vi "Down.vi"(8 "error in (no error)":errorcluster, 11 "Hijo in":refnum<class "Hijo.lvclass">) -> (0 "error out":errorcluster, 3 "Hijo out":refnum<class "Hijo.lvclass">)   [LabVIEW 2020, in "Hijo.lvlib" / "Hijo.lvclass"]
uses:
  Hijo.lvclass
  Hijo.lvclass/Hijo.ctl
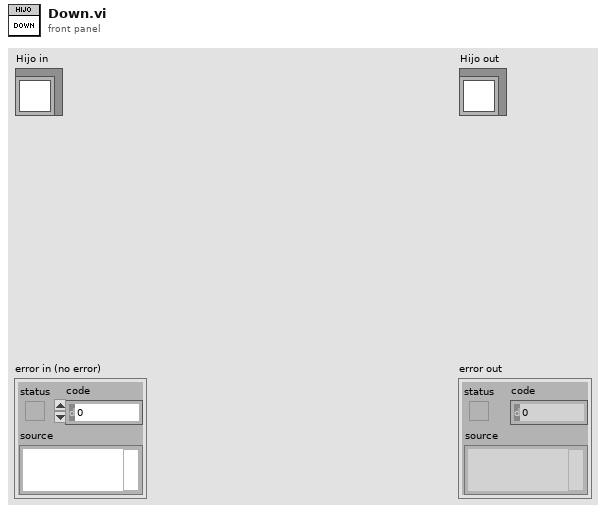
[diagram p1: front panel]
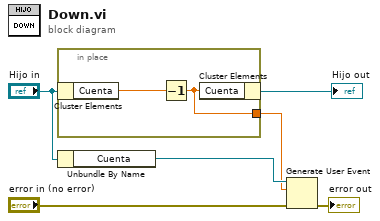
[diagram p0: block diagram]
diagram:
  n1 = in-place {
    in-place-border: [w7] -> w5
    n2 = in-place-cluster #1("Hijo in") -> ("Cuenta"=w8:dbl)
    n3 = Decrement(x=w8) -> (x-1=w7:dbl)
    n4 = in-place-cluster #1("Cuenta"=w7) -> (→"Hijo out":refnum<class "Hijo.lvclass">)
  }
  n5 = Unbundle By Name("Hijo in") -> ("Cuenta"=w6:refnum<user-event>)
  n6 = Generate User Event(user event=w6, event data cluster=w5, error in="error in (no error)") -> (error out=→"error out":errorcluster)  [unwired: 1 in, 1 out]
